vi "Audio_Thread.vi"(9 "channel":T1, 10 "Volume":dbl, 11 "Digital in":refnum<vi>) -> (3 "Audio Loop Time":dbl=0.009959866499998497 format="%#_3ps")   [LabVIEW 2020]
uses:
  <extravilib>/ChannelInstances/High Speed Stream-a[.](sgl)/)Channel.ctl
  <vilib>/sound2/lvsound2.llb/Sound Data Format.ctl
  <vilib>/sound2/lvsound2.llb/Sampling Mode.ctl
  7eb1333e-139c-4586-ad35-70723bb5114f.vi
  <extravilib>/ChannelInstances/High Speed Stream-a[.](sgl)/_Read For Replicate.vi
  <extravilib>/ChannelInstances/High Speed Stream-a[.](sgl)/)Channel.vi
  <extravilib>/ChannelInstances/High Speed Stream-a[.](sgl)/Abort Signal/Init Signal.vi
  <vilib>/sound2/lvsound2.llb/Sound Output Write (DBL Single).vi
  <vilib>/ptbypt/NI_PtbyPt.lvlib
  bfbe7921-60db-4d7c-a18c-8dfaaaada73c.vi
  <vilib>/Dataflow_G/G-Audio/G-Audio.lvlib
  <vilib>/Dataflow_G/G-Audio/Controls/Backends.ctl
  <vilib>/Dataflow_G/G-Audio/Controls/Audio Device Format.ctl
  <vilib>/Dataflow_G/G-Audio/Controls/Audio Device Config.ctl
  54a698ef-2469-4f61-9ca4-d890702b7867.vi
  <extravilib>/ChannelInstances/High Speed Stream-a[.](sgl).lvlib
panel:
  out "Audio Loop Time 2":dbl=0.009959866499998497 format="%#_3ps"
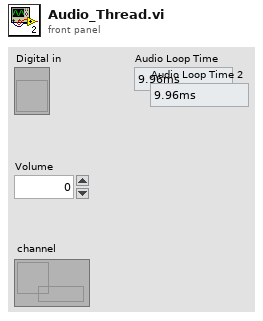
[diagram p1: front panel]
types:
  T1 = typedef "High Speed Stream-a[.](sgl).lvlib/)Channel.ctl" = refnum<queue>
  T2 = typedef "G-Audio.lvlib/Audio Device Config.ctl" = cluster{"Sample Rate (Hz)":u32, "Channels":u32, "Format":T3}
  T3 = typedef "G-Audio.lvlib/Audio Device Format.ctl" = enum16{"Native", "U8", "I16", "I32", "SGL"}
  T4 = typedef "G-Audio.lvlib/Backends.ctl" = enum16{"WASAPI", "DirectSound", "WinMM", "Core Audio", "sndio", "audio(4)", "OSS", "PulseAudio", "ALSA", "JACK", "AAudio", "OpenSL|ES", "Web Audio", "Custom", "Null", "Default"}
  T5 = typedef "Sound Data Format.ctl" = cluster{"sample rate (S/s)":dbl, "number of channels":i32, "bits per sample":i32}
  T6 = typedef "Sampling Mode.ctl" = i32
  T7 = typedef "Sound Output Task ID.ctl" = u32
  T8 = typedef "G-Audio.lvlib/Audio Device Refnum.ctl" = refnum<file>
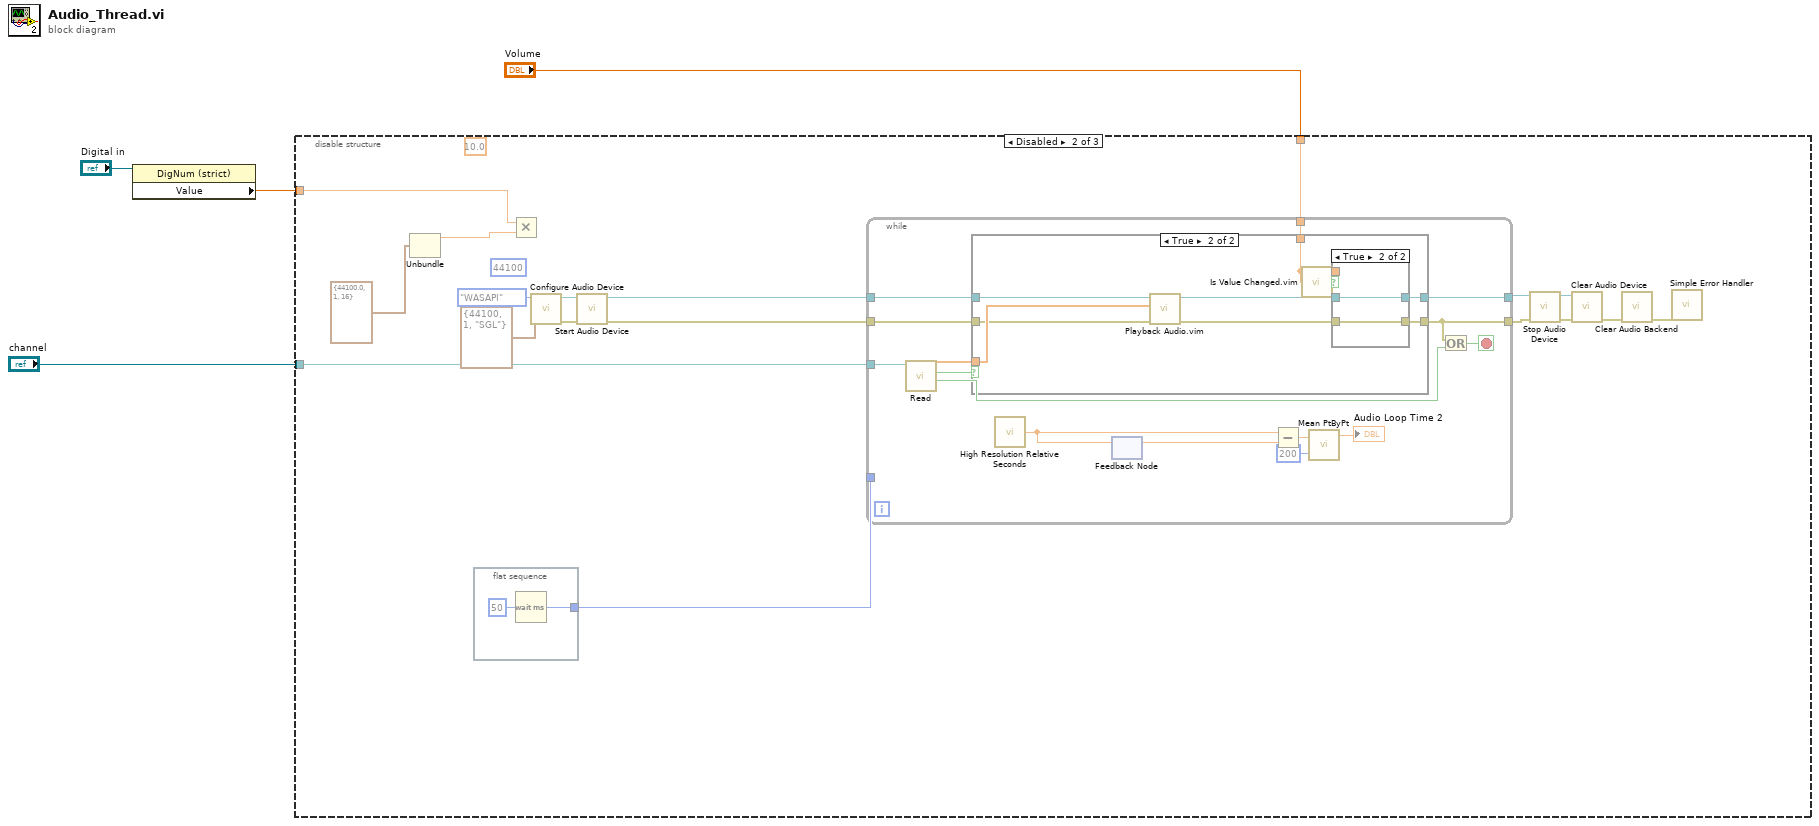
[diagram p0: block diagram]
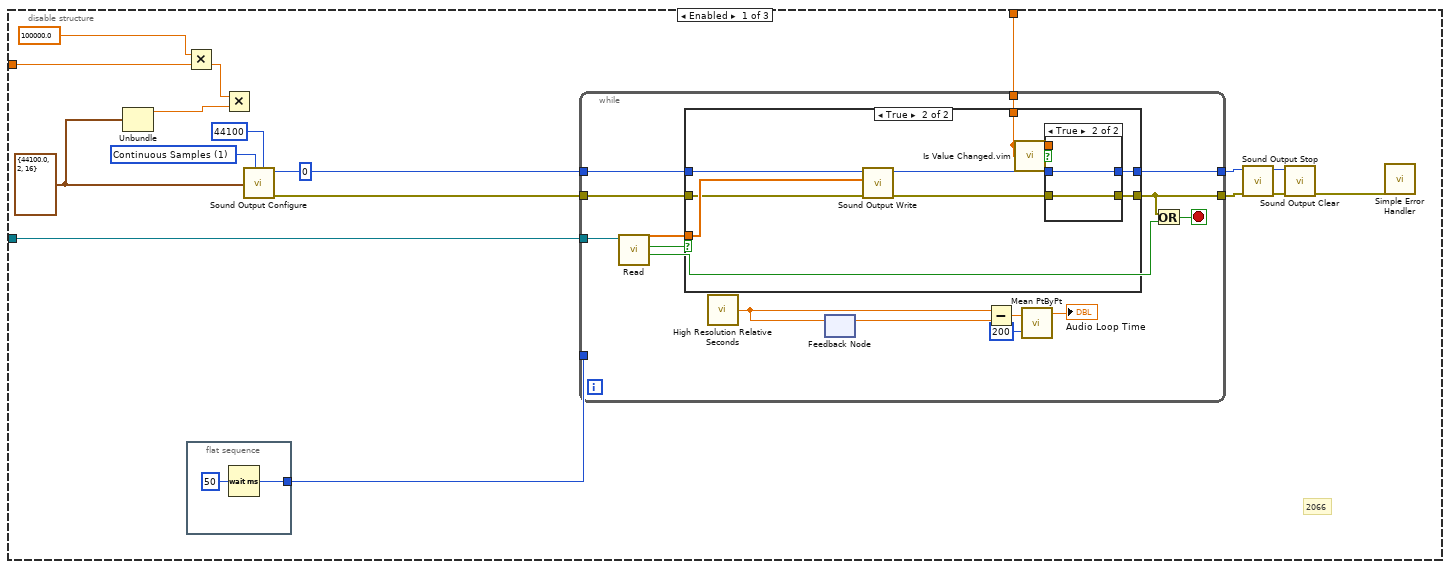
[diagram p2: hidden frame]
diagram:
  n1 = property class="DigNum (strict)"(reference="Digital in") -> ("Value"=w2:dbl)  [unwired: 1 in, 2 out]
  n2 = disable-structure shown="Disabled" {
    disable-tunnel: "channel" -> [w22 w72 _]
    disable-tunnel: "Volume" -> [w21 w71 _]
    disable-tunnel: w2 -> [w8 w62 _]
    frame Enabled {
      w14 = T5 {"sample rate (S/s)"=44100.0, "number of channels"=2, "bits per sample"=16} ("Public Parameters.sound format")
      w13 = T6 1 items=["Finite Samples", "Continuous Samples"] ("Public Parameters.sample mode")
      # "2066"
      n3 = Unbundle(w14) -> ("sample rate (S/s)"=w15:dbl)  [unwired: 2 out]
      n4 = Multiply(x=100000.0, y=w8) -> (x*y=w7:dbl)
      n5 = flat-sequence {
        tunnel: [w23] -> w20
        frame #0 {
          n6 = Wait (ms)(milliseconds to wait=u32 50) -> (millisecond timer value=w23:u32)
        }
      }
      n7 = Multiply(x=w7, y=w15) -> ()  [unwired: 1 out]
      n8 = call <vilib>:"Sound Output Configure.vi"("number of samples/ch"=44100, "sample mode"=w13, "sound format"=w14, "device ID"=u32 0 ("Public Parameters.device ID")) -> ("error out"=w19:errorcluster, "task ID"=w17:T7)  [unwired: 3 in, 3 out]
      n9 = while {
        tunnel: w22 -> [w39]
        tunnel: [w36] -> w16
        tunnel: w17 -> [w35]
        tunnel: [w27] -> w18
        tunnel: w19 -> [w26]
        tunnel: w20 -> [_]
        tunnel: w21 -> [w25]
        stop <- w38 stop-if-true
        n10 = call <extravilib>:"Read.vi"("channel"=w39) -> ("done?"=w37:bool, "element valid?"=w34:bool, "element"=w29:sgl[])  [unwired: 6 in, 2 out]
        n11 = case shown="True" w34 {
          tunnel: [w41 w50] -> w36
          tunnel: w35 -> [w41 w49]
          tunnel: w29 -> [_ w48]
          tunnel: [w40 w47] -> w27
          tunnel: w26 -> [w40 w46]
          tunnel: w25 -> [_ w45]
          frame False {
          }
          frame True {
            n12 = call-poly <vilib>:"Sound Output Write.vi"("error in (no error)"=w46, "data"=w48, "task ID"=w49) -> ("error out"=w43:errorcluster, "task ID out"=w42:T7)  [unwired: 7 in]
            n13 = call "Is Value Changed.vim"("value"=w45) -> ("changed or first call?"=w44:bool)
            n14 = case shown="True" w44 {
              tunnel: [w52 w54] -> w50
              tunnel: w42 -> [w52 w54]
              tunnel: w43 -> [w51 w53]
              tunnel: w45 -> [_ _]
              tunnel: [w51 w53] -> w47
              frame False {
              }
              frame True {
              }
            }
          }
        }
        n15 = call <vilib>:"High Resolution Relative Seconds.vi"() -> ("relative seconds"=w32:dbl)
        n16 = feedback #1() -> (w33:dbl)  [unwired: 1 in]
        n17 = feedback-in #1(w32) -> ()
        n18 = Subtract(x=w32, y=w33) -> (x-y=w30:dbl)
        n19 = call <vilib>:"Mean PtByPt.vi"("x"=w30, "sample length"=200) -> ("mean"=→"Audio Loop Time":dbl)  [unwired: 2 in, 1 out]
        n20 = Or(x=w27, y=w37) -> (x .or. y?=w38:bool)
      }
      n21 = call <vilib>:"Sound Output Stop.vi"("error in (no error)"=w18, "task ID"=w16) -> ("error out"=w9:errorcluster, "task ID out"=w10:T7)  [unwired: 8 in]
      n22 = call <vilib>:"Sound Output Clear.vi"("error in (no error)"=w9, "task ID"=w10) -> ("error out"=w11:errorcluster)  [unwired: 9 in]
      n23 = call <vilib>:"Simple Error Handler.vi"("error in (no error)"=w11) -> ()  [unwired: 4 in, 5 out]
    }
    frame Disabled {
      (unwired) 44100 ("Buffer Size (4096)")
      (unwired) 10.0 ("x")
      n24 = Unbundle(T5 {"sample rate (S/s)"=44100.0, "number of channels"=1, "bits per sample"=16} ("Public Parameters.sound format")) -> ("sample rate (S/s)"=w67:dbl)  [unwired: 2 out]
      n25 = flat-sequence {
        tunnel: [w73] -> w70
        frame #0 {
          n26 = Wait (ms)(milliseconds to wait=u32 50) -> (millisecond timer value=w73:u32)
        }
      }
      n27 = Multiply(x=w62, y=w67) -> ()  [unwired: 1 out]
      n28 = call <vilib>:"Configure Audio Device.vi"("Device Config"=T2 {"Sample Rate (Hz)"=44100, "Channels"=1, "Format"=enum."SGL"}, "Backend (Default)"=Backends."WASAPI") -> ("error out"=w69:errorcluster, "Audio Device Refnum"=w58:T8)  [unwired: 6 in, 2 out]
      n29 = call <vilib>:"Start Audio Device.vi"("error in (no error)"=w69, "Audio Device Refnum In"=w58) -> ("error out"=w59:errorcluster, "Audio Device Refnum Out"=w57:T8)  [unwired: 8 in]
      n30 = while {
        tunnel: w72 -> [w89]
        tunnel: [w86] -> w56
        tunnel: w57 -> [w85]
        tunnel: [w77] -> w68
        tunnel: w59 -> [w76]
        tunnel: w70 -> [_]
        tunnel: w71 -> [w75]
        stop <- w88 stop-if-true
        n31 = call <extravilib>:"Read.vi"("channel"=w89) -> ("done?"=w87:bool, "element valid?"=w84:bool, "element"=w79:sgl[])  [unwired: 6 in, 2 out]
        n32 = case shown="True" w84 {
          tunnel: [w91 w92] -> w86
          tunnel: w85 -> [w91 w93]
          tunnel: w79 -> [_ w100]
          tunnel: [w90 w99] -> w77
          tunnel: w76 -> [w90 w98]
          tunnel: w75 -> [_ w97]
          frame False {
          }
          frame True {
            n33 = call "Playback Audio.vim"("error in (no error)"=w98, "Audio Data"=w100, "Audio Device Refnum In"=w93) -> ("error out"=w94:errorcluster, "Audio Device Refnum Out"=w95:T8)  [unwired: 7 in]
            n34 = call "Is Value Changed.vim"("value"=w97) -> ("changed or first call?"=w96:bool)
            n35 = case shown="True" w96 {
              tunnel: [w102 w103] -> w92
              tunnel: w95 -> [w102 w103]
              tunnel: w94 -> [w101 w104]
              tunnel: w97 -> [_ _]
              tunnel: [w101 w104] -> w99
              frame False {
              }
              frame True {
              }
            }
          }
        }
        n36 = call <vilib>:"High Resolution Relative Seconds.vi"() -> ("relative seconds"=w82:dbl)
        n37 = feedback #2() -> (w83:dbl)  [unwired: 1 in]
        n38 = feedback-in #2(w82) -> ()
        n39 = Subtract(x=w82, y=w83) -> (x-y=w80:dbl)
        n40 = call <vilib>:"Mean PtByPt.vi"("x"=w80, "sample length"=200) -> ("mean"=→"Audio Loop Time 2":dbl)  [unwired: 2 in, 1 out]
        n41 = Or(x=w77, y=w87) -> (x .or. y?=w88:bool)
      }
      n42 = call <vilib>:"Stop Audio Device.vi"("error in (no error)"=w68, "Audio Device Refnum In"=w56) -> ("error out"=w63:errorcluster, "Audio Device Refnum Out"=w64:T8)  [unwired: 8 in]
      n43 = call <vilib>:"Clear Audio Device.vi"("error in (no error)"=w63, "Audio Device Refnum In"=w64) -> ("error out"=w65:errorcluster)  [unwired: 9 in]
      n44 = call <vilib>:"Clear Audio Backend.vi"("error in (no error)"=w65) -> ("error out"=w55:errorcluster)  [unwired: 10 in]
      n45 = call <vilib>:"Simple Error Handler.vi"("error in (no error)"=w55) -> ()  [unwired: 4 in, 5 out]
    }
    frame Disabled {
    }
  }
